vi "Select Physical Channels.vi"(8 "error in":errorcluster, 11 "Physical Channels In":bool[](array[boolean])) -> (0 "error out":errorcluster, 2 "Cancelled?":bool, 3 "Physical Channels Out":bool[](array[boolean]))   [LabVIEW 2020, in "NI PXIe-4340 System Explorer.lvlib"]
doc: "When called, launches a dialogue to select AO channels to be added to the system definition"
uses:
  NI PXIe-4340 System Explorer.lvlib
panel:
  in  "Tree":string(tree)
  in  "Cancel":bool
  in  "Accept":bool
  # "Please Select the Channels to Use"
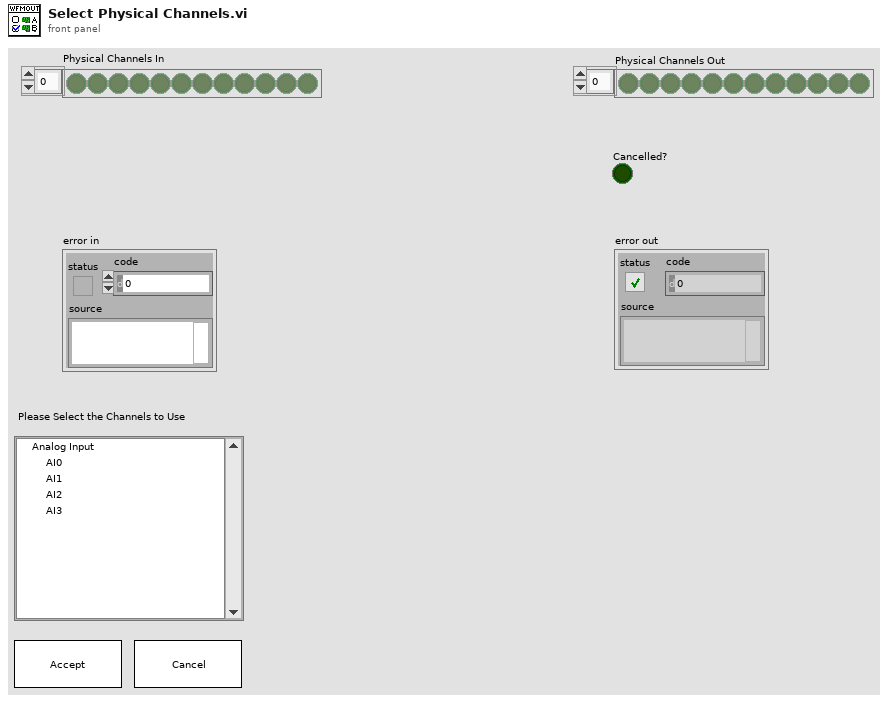
[diagram p1: front panel]
types:
  T1 = typedef "LVPoint32TypeDef.ctl" = cluster{"Horizontal":i32, "Vertical":i32}
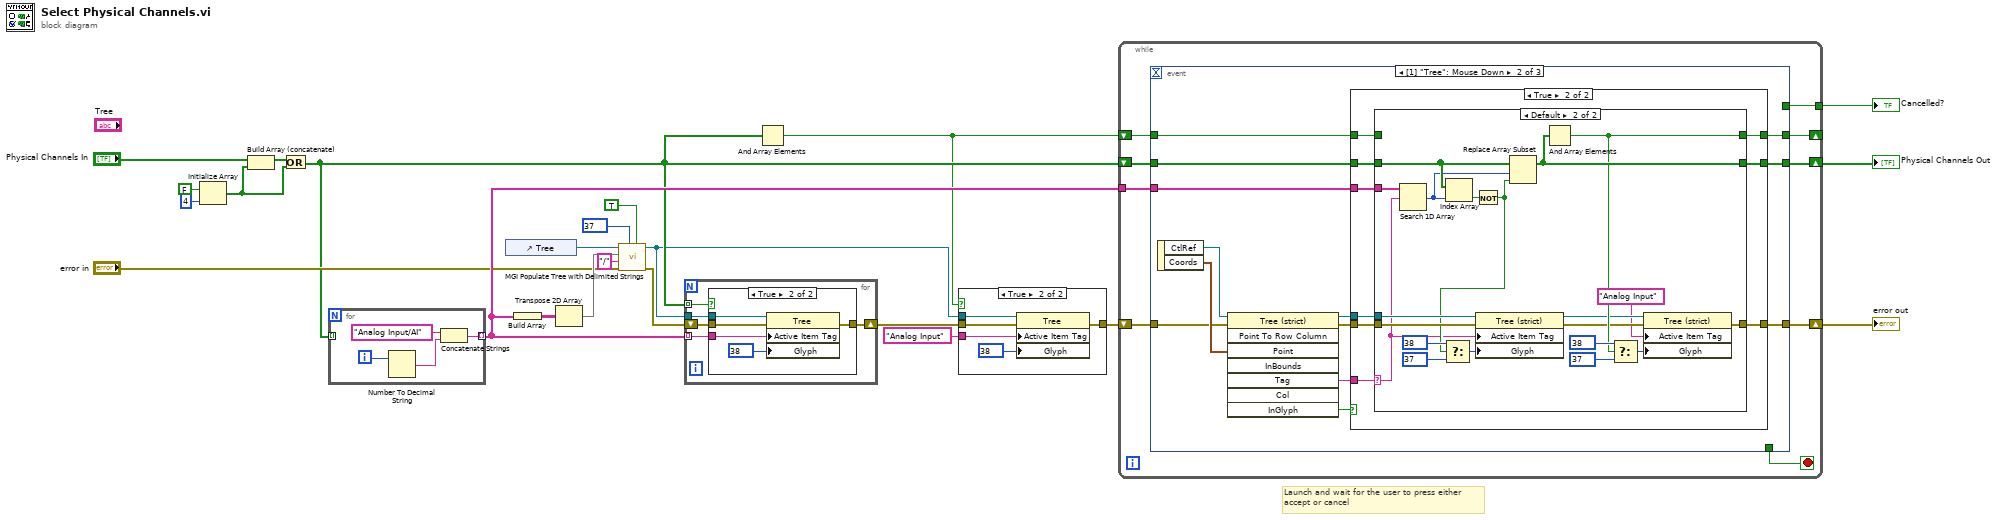
[diagram p0: block diagram]
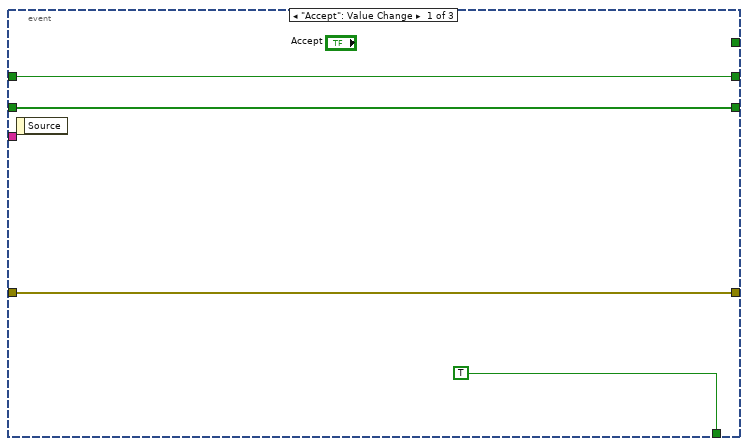
[diagram p4: hidden frame]
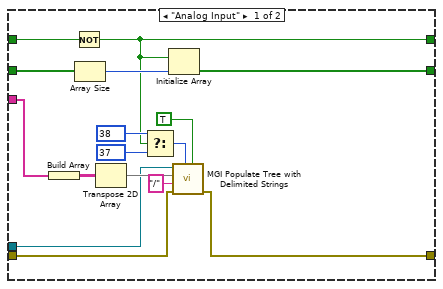
[diagram p6: hidden frame]
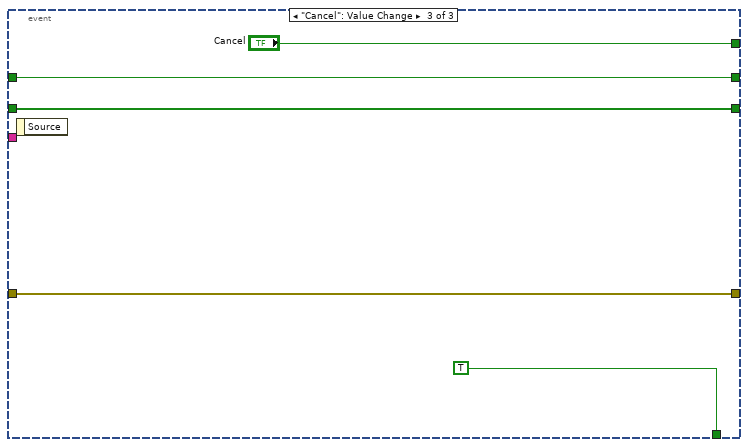
[diagram p7: hidden frame]
diagram:
  # "Launch and wait for the user to press either\naccept or cancel"
  n1 = Initialize Array(FALSE, 4 ("dimension size")) -> (w9:bool[])
  n2 = Build Array (concatenate)("Physical Channels In", w9) -> (w11:bool[])
  n3 = Or(x=w11, y=w9) -> (x .or. y?=w6:bool[])
  n4 = for {
    tunnel: [w24] -> w14 mode=indexing
    tunnel: w6 -> [_] mode=indexing
    i -> [w27]
    n5 = Number To Decimal String(number=w27) -> (decimal integer string=w26:string)  [unwired: 1 in]
    n6 = Concatenate Strings("Analog Input/AI" ("string"), w26) -> (w24:string)
  }
  n7 = control-ref of="Tree"() -> (w21:refnum<vi>)
  n8 = Build Array(w14) -> (w18:string[][])
  n9 = Transpose 2D Array(2D array=w18) -> (transposed array=w16:string[][])
  n10 = call <userlib>:"MGI Populate Tree with Delimited Strings.vi"("Use Child Only?"=TRUE, "Default Symbol"=37, "error in (no error)"="error in", "Delimiter"="/", "Items (Delimited)"=w16, "Tree Control"=w21) -> ("error out"=w15:errorcluster, "Tree Control Dup"=w4:refnum<vi>)  [unwired: 3 in, 1 out]
  n11 = for {
    tunnel: w14 -> [w31] mode=indexing
    tunnel: w6 -> [w30] mode=indexing
    shift-right: [w28] -> w3
    shift-left: w15 -> [w29]
    tunnel: w4 -> [w32]
    n12 = case shown="True" w30 {
      tunnel: w32 -> [_ w38]
      tunnel: w31 -> [_ w37]
      tunnel: w29 -> [w33 w35]
      tunnel: [w33 w34] -> w28
      frame False {
      }
      frame True {
        n13 = property class="Tree"(reference=w38, error in=w35, "Active Item Tag"=w37, "Glyph"=38) -> (error out=w34:errorcluster)  [unwired: 1 out]
      }
    }
  }
  n14 = And Array Elements(Boolean array=w6) -> (logical AND=w5:bool)
  n15 = case shown="True" w5 {
    tunnel: w4 -> [_ w44]
    tunnel: "Analog Input" ("Active Item:Tag") -> [_ w43]
    tunnel: w3 -> [w39 w41]
    tunnel: [w39 w40] -> w2
    frame False {
    }
    frame True {
      n16 = property class="Tree"(reference=w44, error in=w41, "Active Item Tag"=w43, "Glyph"=38) -> (error out=w40:errorcluster)  [unwired: 1 out]
    }
  }
  n17 = while {
    tunnel: [w52] -> w22
    shift-right: [w53] -> w23
    shift-left: w6 -> [w51]
    shift-right: [w48] -> w13
    shift-left: w2 -> [w49]
    tunnel: w14 -> [w47]
    shift-right: [w45] -> _
    shift-left: w5 -> [w46]
    stop <- w50 stop-if-true
    n18 = event shown="[1] \"Tree\": Mouse Down" {
      selector: _ -> [_ _ _]
      dyn-events: _ -> [_ _ _]
      timeout: _ -> [_ _ _]
      tunnel: [w55 w65 w123] -> w53
      tunnel: w51 -> [w55 w64 w123]
      tunnel: [_ _ "Cancel"] -> w52
      tunnel: [TRUE _ TRUE] -> w50
      tunnel: w49 -> [w56 w67 w120]
      tunnel: [w56 w63 w120] -> w48
      tunnel: w47 -> [_ w61 _]
      tunnel: w46 -> [w54 w60 w119]
      tunnel: [w54 w59 w119] -> w45
      event "Accept": Value Change {
        n19 = event-data() -> ()  [unwired: 1 in, 1 out]
      }
      event "Tree": Mouse Down {
        n20 = event-data() -> ("CtlRef"=w58:refnum<vi>, "Coords"=w70:T1)  [unwired: 1 in]
        n21 = invoke class="Tree (strict)" method="Point To Row Column"(reference=w58, error in=w67, "Point"=w70) -> (reference out=w69:refnum<vi>, error out=w66:errorcluster, "Tag"=w68:string, "InGlyph"=w62:bool)  [unwired: 5 in, 4 out]
        n22 = case shown="True" w62 {
          tunnel: w69 -> [_ w82]
          tunnel: w68 -> [_ w76]
          tunnel: w66 -> [w72 w81]
          tunnel: [w73 w78] -> w65
          tunnel: w64 -> [w73 w77]
          tunnel: [w72 w80] -> w63
          tunnel: w61 -> [_ w79]
          tunnel: w60 -> [w71 w75]
          tunnel: [w71 w74] -> w59
          frame False {
          }
          frame True {
            n23 = case shown="Default" w76 {
              selector: w76 -> [_ w108]
              tunnel: w82 -> [w83 w118]
              tunnel: w81 -> [w85 w117]
              tunnel: [w84 w100] -> w80
              tunnel: w79 -> [w86 w116]
              tunnel: [w95 w107] -> w78
              tunnel: w77 -> [w97 w115]
              tunnel: w75 -> [w98 _]
              tunnel: [w92 w103] -> w74
              frame "Analog Input" {
                n24 = Build Array(w86) -> (w89:string[][])
                n25 = Not(x=w98) -> (.not. x?=w92:bool)
                n26 = Array Size(array=w97) -> (size(s)=w96:i32)
                n27 = Transpose 2D Array(2D array=w89) -> (transposed array=w91:string[][])
                n28 = Select(t=38, s=w92, f=37) -> (s? t:f=w87:i32)
                n29 = Initialize Array(w92, w96) -> (w95:bool[])
                n30 = call <userlib>:"MGI Populate Tree with Delimited Strings.vi"("Use Child Only?"=TRUE, "Default Symbol"=w87, "error in (no error)"=w85, "Delimiter"="/", "Items (Delimited)"=w91, "Tree Control"=w83) -> ("error out"=w84:errorcluster)  [unwired: 3 in, 2 out]
              }
              frame Default {
                n31 = Search 1D Array(1D array=w116, element=w108) -> (index of element=w113:i32)  [unwired: 1 in]
                n32 = Index Array(array=w115, index=w113) -> (element=w114:bool)
                n33 = Not(x=w114) -> (.not. x?=w109:bool)
                n34 = Select(t=38, s=w109, f=37) -> (s? t:f=w110:i32)
                n35 = property class="Tree (strict)"(reference=w118, error in=w117, "Active Item Tag"=w108, "Glyph"=w110) -> (reference out=w101:refnum<vi>, error out=w102:errorcluster)
                n36 = Replace Array Subset(array=w115, new element=w109, index=w113) -> (w107:bool[])
                n37 = And Array Elements(Boolean array=w107) -> (logical AND=w103:bool)
                n38 = Select(t=38, s=w103, f=37) -> (s? t:f=w106:i32)
                n39 = property class="Tree (strict)"(reference=w101, error in=w102, "Active Item Tag"="Analog Input" ("Active Item:Tag"), "Glyph"=w106) -> (error out=w100:errorcluster)  [unwired: 1 out]
              }
            }
          }
        }
      }
      event "Cancel": Value Change {
        n40 = event-data() -> ()  [unwired: 1 in, 1 out]
      }
    }
  }
  "Physical Channels Out" <- w23
  "Cancelled?" <- w22
  "error out" <- w13
